vi "Page_Source_Initialize.vi"(8 "error in (no error)":errorcluster, 9 "ctlReferences":T1, 11 "AB_InteropAssembly in":refnum<class "AB_InteropAssembly.lvclass">) -> (0 "error out":errorcluster, 1 "supportedFunctions":T2, 3 "AB_InteropAssembly out":refnum<class "AB_InteropAssembly.lvclass">)   [LabVIEW 2020, in "AB_InteropAssembly.lvclass"]
uses:
  <vilib>/AppBuilder/AB_Classes/InteropAssembly/AB_InteropAssembly.lvclass
  <resource>/Framework/Providers/Builds/AppBuilder/AB_UI_Page_Source_Files_supportedFunctions.ctl
  <vilib>/AppBuilder/AB_Source_Inclusion.ctl
  <resource>/Framework/Providers/Builds/AppBuilder/AB_UI_Page_Source_Files_References.ctl
  <resource>/Framework/Providers/Common/provcom_StringGlobals.vi
  <vilib>/AppBuilder/AB_Classes/Application/AB_Application.lvclass
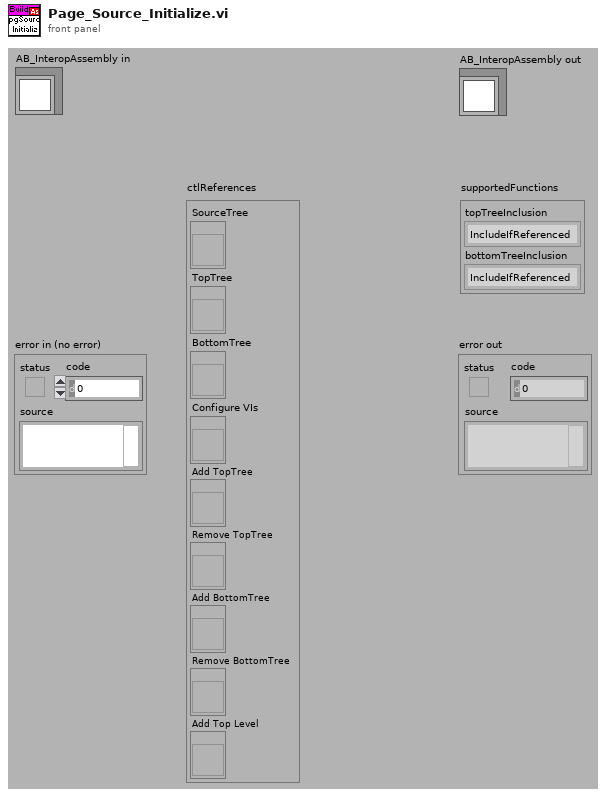
[diagram p1: front panel]
types:
  T1 = typedef "AB_UI_Page_Source_Files_References.ctl" = cluster{"SourceTree":refnum<vi>, "TopTree":refnum<vi>, "BottomTree":refnum<vi>, "Configure VIs":refnum<vi>, "Add TopTree":refnum<vi>, "Remove TopTree":refnum<vi>, "Add BottomTree":refnum<vi>, "Remove BottomTree":refnum<vi>, "Add Top Level":refnum<vi>}
  T2 = typedef "AB_UI_Page_Source_Files_supportedFunctions.ctl" = cluster{"topTreeInclusion":T3, "bottomTreeInclusion":T3}
  T3 = typedef "AB_Source_Inclusion.ctl" = enum16{"IncludeIfReferenced", "Include", "Exclude", "TopLevel"}
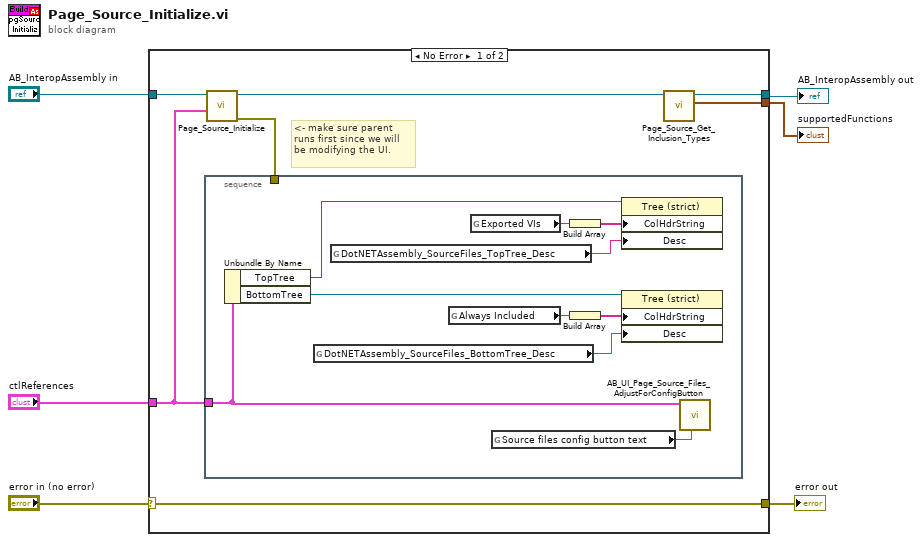
[diagram p0: block diagram]
diagram:
  n1 = case shown="No Error" "error in (no error)" {
    selector: "error in (no error)" -> [w11 w25]
    tunnel: [w11 w25] -> w4
    tunnel: "AB_InteropAssembly in" -> [w10 w24]
    tunnel: "ctlReferences" -> [w7 _]
    tunnel: [w12 _] -> w5
    tunnel: [w13 w24] -> w1
    frame No Error {
      # "<- make sure parent runs first since we will be modifying the UI."
      n2 = call-parent "Page_Source_Initialize.vi"("ctlReferences"=w7, "AB_Build in"=w10) -> ("error out"=w8:errorcluster, "AB_Build out"=w9:refnum<class "AB_InteropAssembly.lvclass">)  [unwired: 7 in, 1 out]
      n3 = stacked-sequence {
        tunnel: w7 -> [w17]
        tunnel: w8 -> [_]
        frame #0 {
          n4 = Unbundle By Name(w17) -> ("TopTree"=w19:refnum<vi>, "BottomTree"=w18:refnum<vi>)
          n5 = global read "provcom_StringGlobals.vi" "DotNETAssembly_SourceFiles_BottomTree_Desc"() -> (w14:string)
          n6 = global read "provcom_StringGlobals.vi" "DotNETAssembly_SourceFiles_TopTree_Desc"() -> (w15:string)
          n7 = global read "provcom_StringGlobals.vi" "Always Included"() -> (w23:string)
          n8 = global read "provcom_StringGlobals.vi" "Exported VIs"() -> (w22:string)
          n9 = global read "provcom_StringGlobals.vi" "Source files config button text"() -> (w16:string)
          n10 = Build Array(w22) -> (w21:string[])
          n11 = Build Array(w23) -> (w20:string[])
          n12 = property class="Tree (strict)"(reference=w19, "ColHdrString"=w21, "Desc"=w15) -> ()  [unwired: 1 in, 2 out]
          n13 = property class="Tree (strict)"(reference=w18, "ColHdrString"=w20, "Desc"=w14) -> ()  [unwired: 1 in, 2 out]
          n14 = call <resource>:"AB_UI_Page_Source_Files_AdjustForConfigButton.vi"("config boolean string"=w16, "ctlReferences"=w17) -> ()  [unwired: 1 in, 9 out]
        }
      }
      n15 = call-dynamic "Page_Source_Get_Inclusion_Types.vi"("AB_InteropAssembly in"=w9) -> ("supportedFunctions"=w12:T2, "AB_InteropAssembly out"=w13:refnum<class "AB_InteropAssembly.lvclass">)  [unwired: 1 in, 8 out]
    }
    frame Error {
    }
  }
  "error out" <- w4
  "supportedFunctions" <- w5
  "AB_InteropAssembly out" <- w1
